vi "Rect Edit.vi"() -> ()   [LabVIEW 2013]
uses:
  Global Variables.vi
panel:
  in  "Index":i32=8
  in  "Direction":u16(ring) items=["Forward", "Backward"]
  in  "Enabled":bool=TRUE
  in  "Voltage Schedule":u16(ring) items=["Constant", "Ramp", "Fn. Generator", "Formula"]
  in  "Apply to All":bool
  in  "Fill Orientation":u16(ring) items=["Horizontal", "Vertical"]
  in  "Speed Schedule":u16(ring) items=["Constant", "Ramp", "Fn. Generator", "Formula"]
  in  "Speed (µm/s)":dbl=8.0
  in  "Voltage (V)":dbl=8.0
  in  "Speed Settings":bool
  in  "Voltage Settings":bool
  in  "Fill Spacing":dbl=0.1
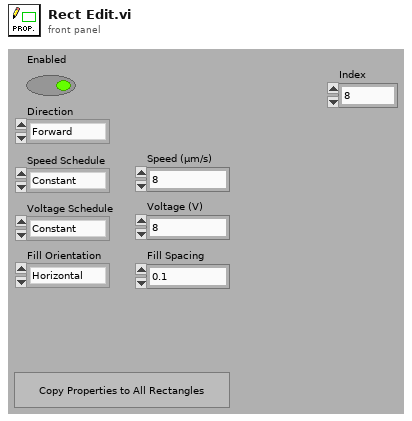
[diagram p1: front panel]
types:
  T1 = enum32{"invalid app kind", "Development System", "Run Time System", "Student Edition", "Embedded LabVIEW", "Evaluation", "Custom"}
  T2 = enum32{"Invalid", "Standard", "Closed", "Hidden", "Minimized", "Maximized"}
  T3 = cluster{"Enabled":bool, "Direction":u16, "Fill Orientation":u16, "Fill Spacing":dbl, "Speed (µm/s)":cluster{"Schedule":u16, "Value":dbl, "Start Value":dbl, "End Value":dbl, "Min Value":dbl, "Max Value":dbl, "Duty Cycle (%)":dbl, "Signal Type":u16, "Cycle Number":dbl, "Phase (degrees)":dbl}, "Voltage (V)":cluster{"Schedule":u16, "Value":dbl, "Start Value":dbl, "End Value":dbl, "Min Value":dbl, "Max Value":dbl, "Duty Cycle (%)":dbl, "Signal Type":u16, "Cycle Number":dbl, "Phase (degrees)":dbl}}[]
  T4 = cluster{"Enabled":bool, "Direction":u16, "Fill Orientation":u16, "Fill Spacing":dbl, "Speed (µm/s)":cluster{"Schedule":u16, "Value":dbl, "Start Value":dbl, "End Value":dbl, "Min Value":dbl, "Max Value":dbl, "Duty Cycle (%)":dbl, "Signal Type":u16, "Cycle Number":dbl, "Phase (degrees)":dbl}, "Voltage (V)":cluster{"Schedule":u16, "Value":dbl, "Start Value":dbl, "End Value":dbl, "Min Value":dbl, "Max Value":dbl, "Duty Cycle (%)":dbl, "Signal Type":u16, "Cycle Number":dbl, "Phase (degrees)":dbl}}
  T5 = cluster{"Schedule":u16, "Value":dbl, "Start Value":dbl, "End Value":dbl, "Min Value":dbl, "Max Value":dbl, "Duty Cycle (%)":dbl, "Signal Type":u16, "Cycle Number":dbl, "Phase (degrees)":dbl}
  T6 = cluster{"Schedule":u16, "Value":dbl, "Start Value":dbl, "End Value":dbl, "Min Value":dbl, "Max Value":dbl, "Duty Cycle (%)":dbl, "Speed Signal Type":u16, "Cycle Number":dbl, "Phase (degrees)":dbl}
  T7 = cluster{"Core":cluster{"Current VI Reference":refnum<vi>, "Close Panel on Exit?":bool}}
  T8 = cluster{"Current VI Reference":refnum<vi>, "Close Panel on Exit?":bool}
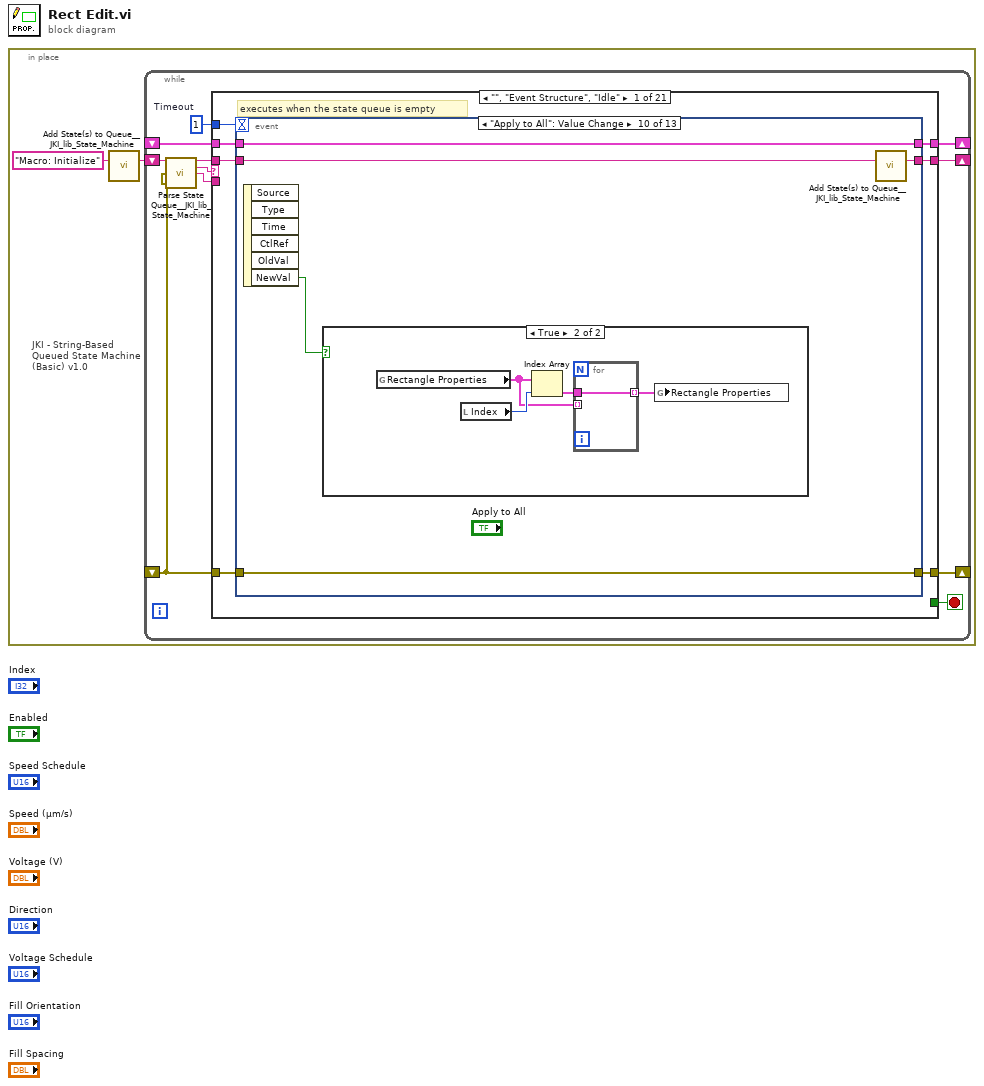
[diagram p0: block diagram]
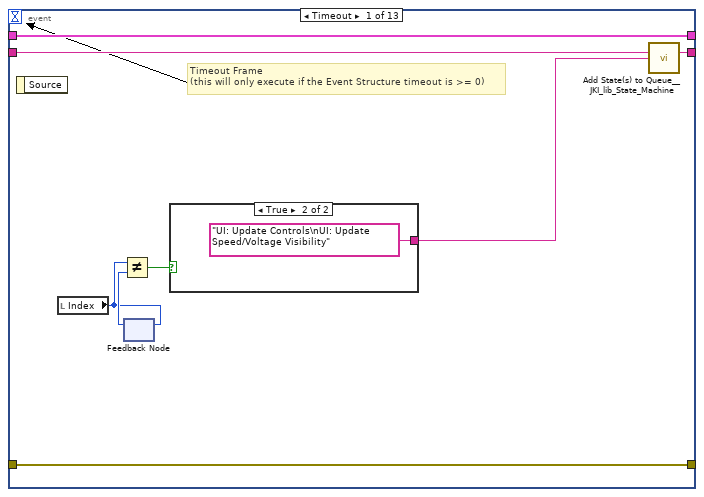
[diagram p2: hidden frame]
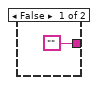
[diagram p3: hidden frame]
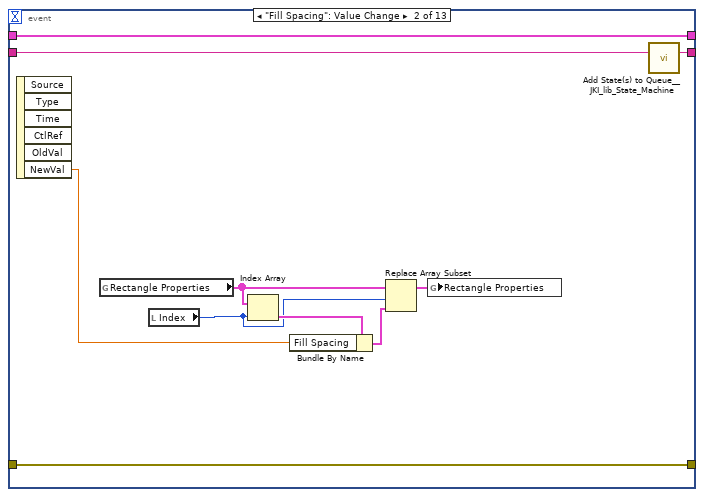
[diagram p4: hidden frame]
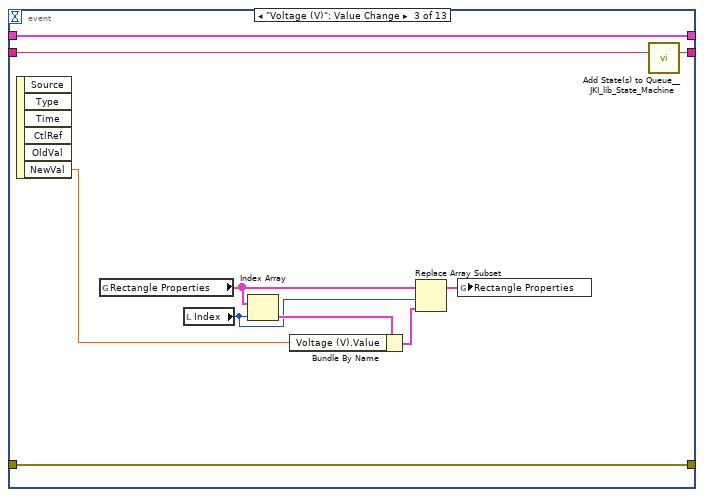
[diagram p5: hidden frame]
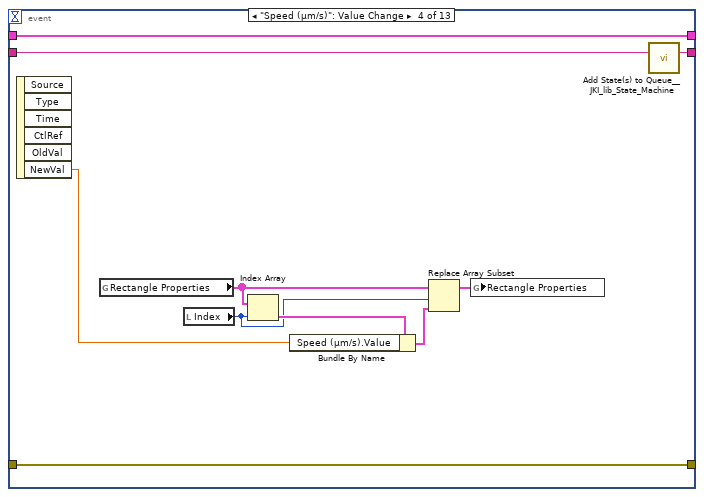
[diagram p6: hidden frame]
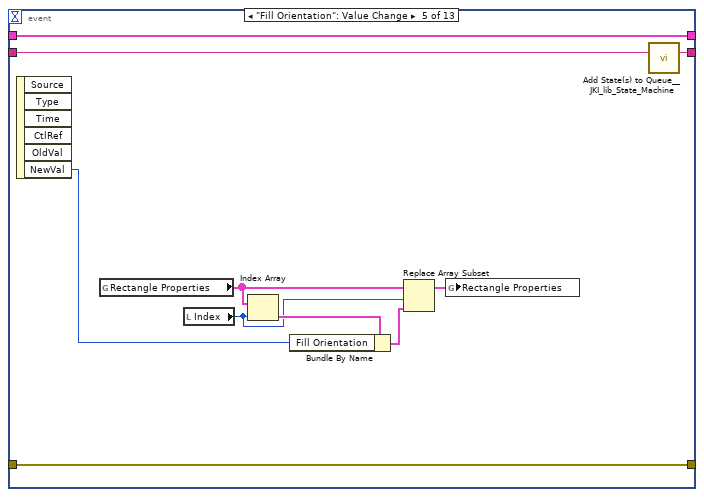
[diagram p7: hidden frame]
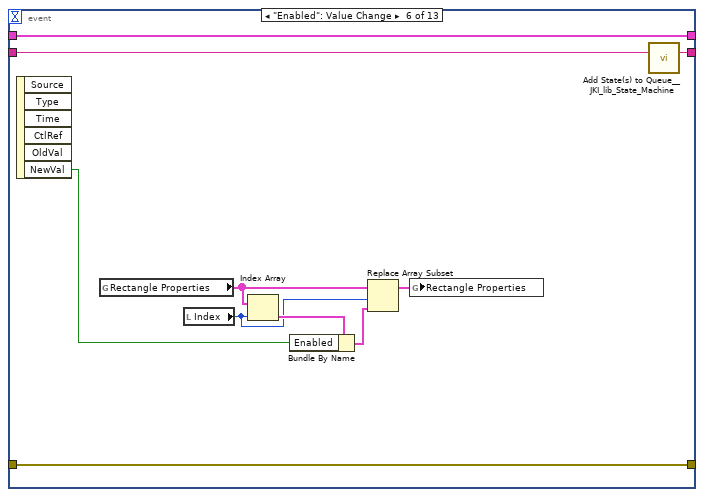
[diagram p8: hidden frame]
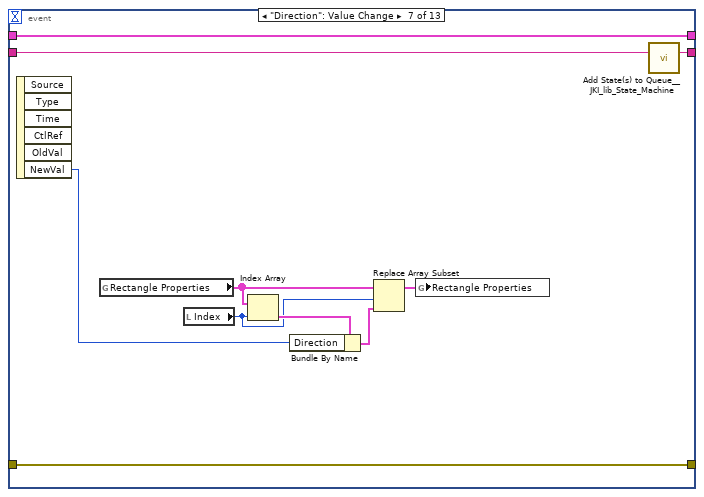
[diagram p9: hidden frame]
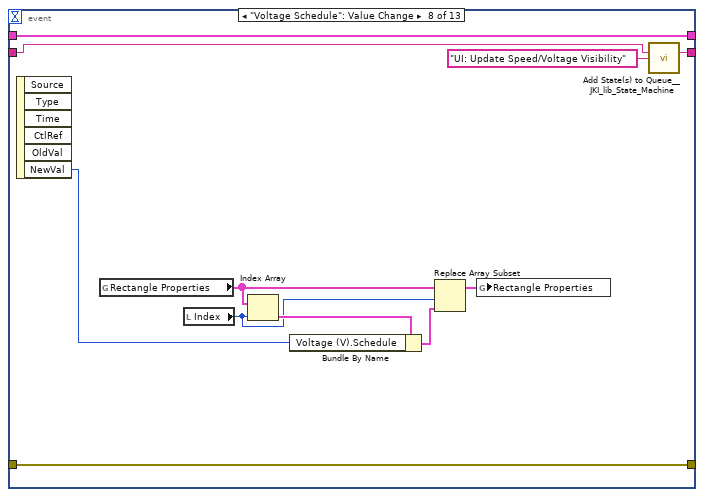
[diagram p10: hidden frame]
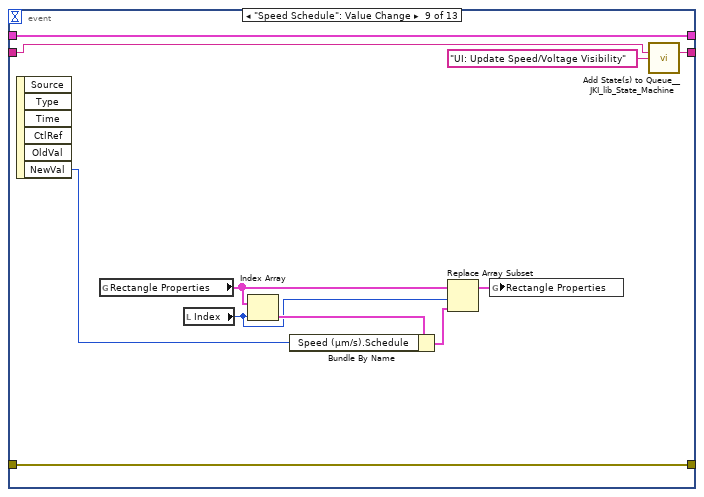
[diagram p11: hidden frame]
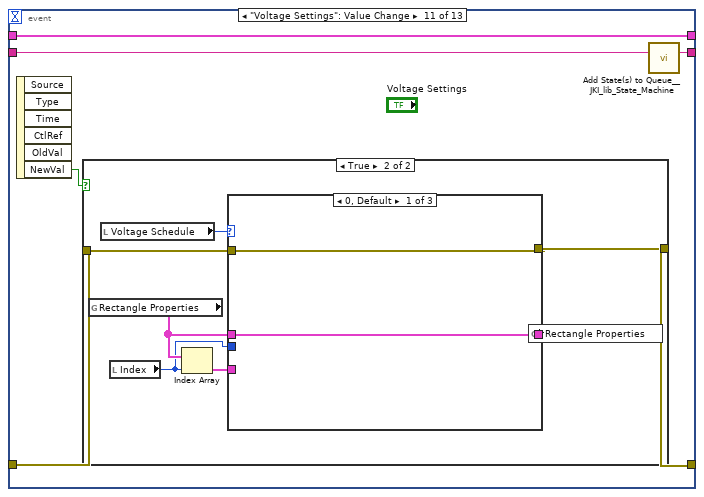
[diagram p13: hidden frame]
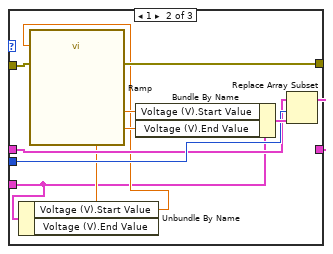
[diagram p15: hidden frame]
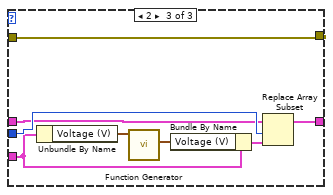
[diagram p16: hidden frame]
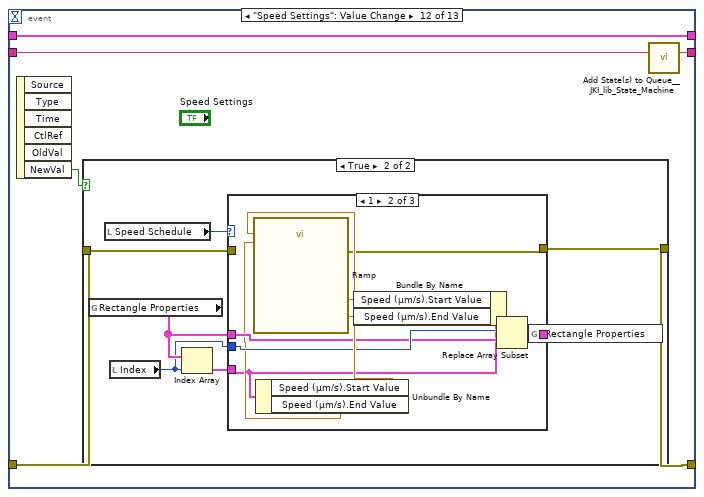
[diagram p17: hidden frame]
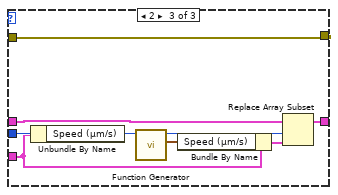
[diagram p20: hidden frame]
diagram:
  n1 = in-place {
    n2 = call <vilib>:"Add State(s) to Queue__JKI_lib_State_Machine.vi"("State(s) in (\"\")"="Macro: Initialize") -> ("States Out"=w2:string)  [unwired: 14 in]
    n3 = while "JKI - String-Based Queued State Machine (Basic) v1.0" {
      shift-right: [w6] -> _
      shift-left: _ -> [w5]
      shift-right: [w9] -> _
      shift-left: _ -> [w3]
      shift-right: [w8] -> _
      shift-left: w2 -> [w10]
      stop <- w7 stop-if-true
      w4 = 1  # Timeout
      n4 = call <vilib>:"Parse State Queue__JKI_lib_State_Machine.vi"("State Queue"=w10, "Error In (no error)"=w3) -> ("Remaining States"=w12:string, "Current State"=w13:string, "Arguments"=w11:string)  [unwired: 11 in]
      n5 = case shown="\"\", \"Event Structure\", \"Idle\"" w13 {
        selector: w13 -> [_ _ w202 _ _ _ _ _ _ _ _ _ _ _ _ _ _ _ _ _ _]
        tunnel: w12 -> [w20 w201 w206 w224 w230 w235 w239 w244 w250 w254 w258 w273 w279 w297 w308 w334 w339 w349 w353 w357 w361]
        tunnel: w11 -> [_ _ _ _ _ _ _ _ _ _ _ _ w274 _ w302 _ _ _ _ _ _]
        tunnel: w5 -> [w18 w198 w204 w220 w227 w233 w236 _ w248 w251 w256 w271 w277 w295 w304 w331 w336 w346 w350 w354 w358]
        tunnel: [w17 w199 w208 w221 errorcluster {"status"=FALSE, "code"=0, "source"=""} ("error out") w232 w237 w240 w246 w252 w255 w260 w275 w284 w305 w332 w337 w347 w351 w355 w359] -> w9
        tunnel: w3 -> [w16 w199 w207 w221 w226 w232 w237 w240 w245 w252 w255 w260 w276 w294 w306 w332 w337 w347 w351 w355 w359]
        tunnel: [w19 w200 w205 w223 w229 w234 w238 w243 w249 w253 w257 w272 w278 w296 w307 w333 w338 w348 w352 w356 w360] -> w8
        tunnel: [_ _ _ _ _ TRUE _ _ _ _ _ _ _ _ _ _ _ _ _ _ _] -> w7
        tunnel: [w15 w198 w204 w222 w227 w233 w236 w242 w248 w251 w256 w271 w277 w295 w304 w331 w336 w346 w350 w354 w358] -> w6
        tunnel: w4 -> [w14 _ _ _ _ _ _ _ _ _ _ _ _ _ _ _ _ _ _ _ _]
        frame "", "Event Structure", "Idle" {
          # "executes when the state queue is empty"
          n6 = event shown="[9] \"Apply to All\": Value Change" {
            selector: _ -> [_ _ _ _ _ _ _ _ _ _ _ _ _]
            dyn-events: _ -> [_ _ _ _ _ _ _ _ _ _ _ _ _]
            timeout: w14 -> [_ _ _ _ _ _ _ _ _ _ _ _ _]
            tunnel: w20 -> [w28 w40 w50 w60 w70 w80 w90 w101 w112 w117 w128 w163 w197]
            tunnel: [w27 w39 w49 w59 w69 w79 w89 w100 w111 w116 w127 w162 w196] -> w19
            tunnel: w18 -> [w25 w38 w48 w58 w68 w78 w88 w99 w110 w115 w126 w161 w194]
            tunnel: [w26 w32 w42 w52 w62 w72 w82 w93 w104 w114 w124 w159 w195] -> w17
            tunnel: w16 -> [w26 w32 w42 w52 w62 w72 w82 w93 w104 w114 w125 w160 w195]
            tunnel: [w25 w38 w48 w58 w68 w78 w88 w99 w110 w115 w126 w161 w194] -> w15
            event Timeout {
              # "Timeout Frame\n(this will only execute if the Event Structure timeout is >= 0)"
              n7 = event-data() -> ()  [unwired: 1 in, 1 out]
              n8 = local read "Index"() -> (w21:i32)
              n9 = feedback #1() -> (w24:i32)  [unwired: 1 in]
              n10 = Not Equal?(x=w21, y=w24) -> (x != y?=w23:bool)
              n11 = feedback-in #1(w21) -> ()
              n12 = case shown="True" w23 {
                tunnel: ["" "UI: Update Controls\nUI: Update Speed/Voltage Visibility"] -> w22
                frame False {
                }
                frame True {
                }
              }
              n13 = call <vilib>:"Add State(s) to Queue__JKI_lib_State_Machine.vi"("State(s) in (\"\")"=w28, "State(s) at Back (\"\")"=w22) -> ("States Out"=w27:string)  [unwired: 13 in]
            }
            event "Fill Spacing": Value Change {
              n14 = event-data() -> ("NewVal"=w36:dbl)  [unwired: 1 in, 5 out]
              n15 = global read "Global Variables.vi" "Rectangle Properties"() -> (w34:T3)
              n16 = local read "Index"() -> (w31:i32)
              n17 = Index Array(array=w34, index=w31) -> (element=w37:T4)
              n18 = Bundle By Name(cluster=w37, "Fill Spacing"=w36) -> (w35:T4)
              n19 = Replace Array Subset(array=w34, new element=w35, index=w31) -> (w33:T3)
              n20 = global write "Global Variables.vi" "Rectangle Properties"(w33) -> ()
              n21 = call <vilib>:"Add State(s) to Queue__JKI_lib_State_Machine.vi"("State(s) in (\"\")"=w40) -> ("States Out"=w39:string)  [unwired: 14 in]
            }
            event "Voltage (V)": Value Change {
              n22 = event-data() -> ("NewVal"=w46:dbl)  [unwired: 1 in, 5 out]
              n23 = global read "Global Variables.vi" "Rectangle Properties"() -> (w44:T3)
              n24 = local read "Index"() -> (w41:i32)
              n25 = Index Array(array=w44, index=w41) -> (element=w47:T4)
              n26 = Bundle By Name(cluster=w47, "Voltage (V).Value"=w46) -> (w45:T4)
              n27 = Replace Array Subset(array=w44, new element=w45, index=w41) -> (w43:T3)
              n28 = global write "Global Variables.vi" "Rectangle Properties"(w43) -> ()
              n29 = call <vilib>:"Add State(s) to Queue__JKI_lib_State_Machine.vi"("State(s) in (\"\")"=w50) -> ("States Out"=w49:string)  [unwired: 14 in]
            }
            event "Speed (µm/s)": Value Change {
              n30 = event-data() -> ("NewVal"=w56:dbl)  [unwired: 1 in, 5 out]
              n31 = global read "Global Variables.vi" "Rectangle Properties"() -> (w54:T3)
              n32 = local read "Index"() -> (w51:i32)
              n33 = Index Array(array=w54, index=w51) -> (element=w57:T4)
              n34 = Bundle By Name(cluster=w57, "Speed (µm/s).Value"=w56) -> (w55:T4)
              n35 = Replace Array Subset(array=w54, new element=w55, index=w51) -> (w53:T3)
              n36 = global write "Global Variables.vi" "Rectangle Properties"(w53) -> ()
              n37 = call <vilib>:"Add State(s) to Queue__JKI_lib_State_Machine.vi"("State(s) in (\"\")"=w60) -> ("States Out"=w59:string)  [unwired: 14 in]
            }
            event "Fill Orientation": Value Change {
              n38 = event-data() -> ("NewVal"=w66:u16)  [unwired: 1 in, 5 out]
              n39 = global read "Global Variables.vi" "Rectangle Properties"() -> (w64:T3)
              n40 = local read "Index"() -> (w61:i32)
              n41 = Index Array(array=w64, index=w61) -> (element=w67:T4)
              n42 = Bundle By Name(cluster=w67, "Fill Orientation"=w66) -> (w65:T4)
              n43 = Replace Array Subset(array=w64, new element=w65, index=w61) -> (w63:T3)
              n44 = global write "Global Variables.vi" "Rectangle Properties"(w63) -> ()
              n45 = call <vilib>:"Add State(s) to Queue__JKI_lib_State_Machine.vi"("State(s) in (\"\")"=w70) -> ("States Out"=w69:string)  [unwired: 14 in]
            }
            event "Enabled": Value Change {
              n46 = event-data() -> ("NewVal"=w76:bool)  [unwired: 1 in, 5 out]
              n47 = global read "Global Variables.vi" "Rectangle Properties"() -> (w74:T3)
              n48 = local read "Index"() -> (w71:i32)
              n49 = Index Array(array=w74, index=w71) -> (element=w77:T4)
              n50 = Bundle By Name(cluster=w77, "Enabled"=w76) -> (w75:T4)
              n51 = Replace Array Subset(array=w74, new element=w75, index=w71) -> (w73:T3)
              n52 = global write "Global Variables.vi" "Rectangle Properties"(w73) -> ()
              n53 = call <vilib>:"Add State(s) to Queue__JKI_lib_State_Machine.vi"("State(s) in (\"\")"=w80) -> ("States Out"=w79:string)  [unwired: 14 in]
            }
            event "Direction": Value Change {
              n54 = event-data() -> ("NewVal"=w86:u16)  [unwired: 1 in, 5 out]
              n55 = global read "Global Variables.vi" "Rectangle Properties"() -> (w84:T3)
              n56 = local read "Index"() -> (w81:i32)
              n57 = Index Array(array=w84, index=w81) -> (element=w87:T4)
              n58 = Bundle By Name(cluster=w87, "Direction"=w86) -> (w85:T4)
              n59 = Replace Array Subset(array=w84, new element=w85, index=w81) -> (w83:T3)
              n60 = global write "Global Variables.vi" "Rectangle Properties"(w83) -> ()
              n61 = call <vilib>:"Add State(s) to Queue__JKI_lib_State_Machine.vi"("State(s) in (\"\")"=w90) -> ("States Out"=w89:string)  [unwired: 14 in]
            }
            event "Voltage Schedule": Value Change {
              n62 = event-data() -> ("NewVal"=w97:u16)  [unwired: 1 in, 5 out]
              n63 = global read "Global Variables.vi" "Rectangle Properties"() -> (w95:T3)
              n64 = local read "Index"() -> (w91:i32)
              n65 = Index Array(array=w95, index=w91) -> (element=w98:T4)
              n66 = Bundle By Name(cluster=w98, "Voltage (V).Schedule"=w97) -> (w96:T4)
              n67 = Replace Array Subset(array=w95, new element=w96, index=w91) -> (w94:T3)
              n68 = global write "Global Variables.vi" "Rectangle Properties"(w94) -> ()
              n69 = call <vilib>:"Add State(s) to Queue__JKI_lib_State_Machine.vi"("State(s) in (\"\")"=w101, "State(s) at Back (\"\")"="UI: Update Speed/Voltage Visibility" ("State(s) at Back (\"\")")) -> ("States Out"=w100:string)  [unwired: 13 in]
            }
            event "Speed Schedule": Value Change {
              n70 = event-data() -> ("NewVal"=w108:u16)  [unwired: 1 in, 5 out]
              n71 = global read "Global Variables.vi" "Rectangle Properties"() -> (w106:T3)
              n72 = local read "Index"() -> (w102:i32)
              n73 = Index Array(array=w106, index=w102) -> (element=w109:T4)
              n74 = Bundle By Name(cluster=w109, "Speed (µm/s).Schedule"=w108) -> (w107:T4)
              n75 = Replace Array Subset(array=w106, new element=w107, index=w102) -> (w105:T3)
              n76 = global write "Global Variables.vi" "Rectangle Properties"(w105) -> ()
              n77 = call <vilib>:"Add State(s) to Queue__JKI_lib_State_Machine.vi"("State(s) in (\"\")"=w112, "State(s) at Back (\"\")"="UI: Update Speed/Voltage Visibility" ("State(s) at Back (\"\")")) -> ("States Out"=w111:string)  [unwired: 13 in]
            }
            event "Apply to All": Value Change {
              n78 = event-data() -> ("NewVal"=w113:bool)  [unwired: 1 in, 5 out]
              n79 = case shown="True" w113 {
                frame False {
                }
                frame True {
                  n80 = global read "Global Variables.vi" "Rectangle Properties"() -> (w118:T3)
                  n81 = local read "Index"() -> (w121:i32)
                  n82 = Index Array(array=w118, index=w121) -> (element=w120:T4)
                  n83 = for {
                    tunnel: w120 -> [w122]
                    tunnel: [w122] -> w119 mode=indexing
                    tunnel: w118 -> [_] mode=indexing
                  }
                  n84 = global write "Global Variables.vi" "Rectangle Properties"(w119) -> ()
                }
              }
              n85 = call <vilib>:"Add State(s) to Queue__JKI_lib_State_Machine.vi"("State(s) in (\"\")"=w117) -> ("States Out"=w116:string)  [unwired: 14 in]
            }
            event "Voltage Settings": Value Change {
              n86 = event-data() -> ("NewVal"=w123:bool)  [unwired: 1 in, 5 out]
              n87 = case shown="True" w123 {
                tunnel: w125 -> [w129 w135]
                tunnel: [w129 w134] -> w124
                frame False {
                }
                frame True {
                  n88 = global read "Global Variables.vi" "Rectangle Properties"() -> (w131:T3)
                  n89 = local read "Voltage Schedule"() -> (w136:u16)
                  n90 = local read "Index"() -> (w130:i32)
                  n91 = Index Array(array=w131, index=w130) -> (element=w132:T4)
                  n92 = case shown="0, Default" w136 {
                    tunnel: w135 -> [w138 w149 w153]
                    tunnel: [w138 w142 w153] -> w134
                    tunnel: [w137 w143 w154] -> w133
                    tunnel: w132 -> [_ w139 w152]
                    tunnel: w131 -> [w137 w144 w155]
                    tunnel: w130 -> [_ w145 w156]
                    frame 0, Default {
                    }
                    frame 1 {
                      n93 = Unbundle By Name(w139) -> ("Voltage (V).Start Value"=w141:dbl, "Voltage (V).End Value"=w140:dbl)
                      n94 = call "Ramp.vi"("Start Value"=w141, "End Value"=w140, "error in (no error)"=w149) -> ("End Value"=w147:dbl, "Start Value"=w148:dbl, "error out"=w142:errorcluster)  [unwired: 13 in, 1 out]
                      n95 = Bundle By Name(cluster=w139, "Voltage (V).Start Value"=w148, "Voltage (V).End Value"=w147) -> (w146:T4)
                      n96 = Replace Array Subset(array=w144, new element=w146, index=w145) -> (w143:T3)
                    }
                    frame 2 {
                      n97 = Unbundle By Name(w152) -> ("Voltage (V)"=w150:T5)
                      n98 = call "Function Generator.vi"("Properties in"=w150) -> ("Properties out"=w151:T6)  [unwired: 9 in, 1 out]
                      n99 = Bundle By Name(cluster=w152, "Voltage (V)"=w151) -> (w157:T4)
                      n100 = Replace Array Subset(array=w155, new element=w157, index=w156) -> (w154:T3)
                    }
                  }
                  n101 = global write "Global Variables.vi" "Rectangle Properties"(w133) -> ()
                }
              }
              n102 = call <vilib>:"Add State(s) to Queue__JKI_lib_State_Machine.vi"("State(s) in (\"\")"=w128) -> ("States Out"=w127:string)  [unwired: 14 in]
            }
            event "Speed Settings": Value Change {
              n103 = event-data() -> ("NewVal"=w158:bool)  [unwired: 1 in, 5 out]
              n104 = case shown="True" w158 {
                tunnel: w160 -> [w164 w170]
                tunnel: [w164 w169] -> w159
                frame False {
                }
                frame True {
                  n105 = global read "Global Variables.vi" "Rectangle Properties"() -> (w166:T3)
                  n106 = local read "Speed Schedule"() -> (w171:u16)
                  n107 = local read "Index"() -> (w165:i32)
                  n108 = Index Array(array=w166, index=w165) -> (element=w167:T4)
                  n109 = case shown="1" w171 {
                    tunnel: w170 -> [w173 _ w187]
                    tunnel: [w173 w179 w187] -> w169
                    tunnel: [w172 w178 w188] -> w168
                    tunnel: w167 -> [_ w174 w186]
                    tunnel: w166 -> [w172 w176 w189]
                    tunnel: w165 -> [_ w177 w190]
                    frame 0, Default {
                    }
                    frame 1 {
                      n110 = Unbundle By Name(w174) -> ("Speed (µm/s).Start Value"=w180:dbl, "Speed (µm/s).End Value"=w175:dbl)
                      n111 = call "Ramp.vi"("Start Value"=w180, "End Value"=w175) -> ("End Value"=w182:dbl, "Start Value"=w183:dbl, "error out"=w179:errorcluster)  [unwired: 14 in, 1 out]
                      n112 = Bundle By Name(cluster=w174, "Speed (µm/s).Start Value"=w183, "Speed (µm/s).End Value"=w182) -> (w181:T4)
                      n113 = Replace Array Subset(array=w176, new element=w181, index=w177) -> (w178:T3)
                    }
                    frame 2 {
                      n114 = Unbundle By Name(w186) -> ("Speed (µm/s)"=w184:T5)
                      n115 = call "Function Generator.vi"("Properties in"=w184) -> ("Properties out"=w185:T6)  [unwired: 9 in, 1 out]
                      n116 = Bundle By Name(cluster=w186, "Speed (µm/s)"=w185) -> (w191:T4)
                      n117 = Replace Array Subset(array=w189, new element=w191, index=w190) -> (w188:T3)
                    }
                  }
                  n118 = global write "Global Variables.vi" "Rectangle Properties"(w168) -> ()
                }
              }
              n119 = call <vilib>:"Add State(s) to Queue__JKI_lib_State_Machine.vi"("State(s) in (\"\")"=w163) -> ("States Out"=w162:string)  [unwired: 14 in]
            }
            event Panel Close? {
              # "Discard the event because we'll close the front panel ourselves in Macro: Exit"
              # "Close Panel button (pressed) Event\n(this executes Macro: Exit to terminate the VI)"
              n120 = event-data() -> ()  [unwired: 1 in, 1 out]
              n121 = event-data("Discard?"=TRUE) -> ()  [unwired: 1 in, 1 out]
              n122 = call <vilib>:"Add State(s) to Queue__JKI_lib_State_Machine.vi"("State(s) in Front (\"\")"="Macro: Exit", "State(s) in (\"\")"=w197) -> ("States Out"=w196:string)  [unwired: 13 in]
            }
          }
        }
        frame "---------- Core ----------" {
          # "Do not put any code in this frame.\n(it is a separator no-op)"
          n123 = call <vilib>:"Add State(s) to Queue__JKI_lib_State_Machine.vi"("State(s) in (\"\")"=w201) -> ("States Out"=w200:string)  [unwired: 14 in]
        }
        frame Default {
          w211 = 42 items=["No error", "Argument error", "Memory is full", "Out of zone", "End of file", "File already open", "Generic file I/O error", "File not found", "File permission error", "Disk is full", "Duplicate path", "Too many files open", "System feature not enabled", "Resource file not found", "Cannot add resource", "Resource not found", "Image not found", "Image memory error", "Pen does not exist", "Config type invalid", "Config token not found", "Config parse error", "Config memory error", "Bad external code format", "Bad external code offset", "External code not present", "Null window", "Destroy window error", "Null menu", "Print aborted", "Bad print record", "Print driver error", "Windows error during printing", "Memory error during printing", "Print dialog error", "Generic print error", "Invalid device refnum", "Device not found", "Device parameter error", "Device unit error", "Cannot open device", "Device call aborted", "Generic error", "Cancelled by user", "Object ID too low", "Object ID too high", "Object not in heap", "Unknown heap", "Unknown object (invalid DefProc)", "Unknown object (DefProc not in table)", "Message out of range", "Invalid (null) method", "Unknown message", "Manager call not supported", "Bad address", "Network operation in progress", "Network operation timed out", "Connection is busy", "Network attribute not supported", "Network error", "Address in use", "System out of memory", "Connection aborted", "Connection refused", "Not connected", "Already connected", "Connection closed", "Initialization error (interapplication manager)", "Bad occurrence", "Wait on unbound occurrence handler", "Occurrence queue overflow", "Datalog type conflict", "Unused", "Unrecognized type (interapplication manager)", "Memory corrupt", "Failed to make temporary DLL", "Old CIN version", "Drag socket not found", "Failed to load drop-object", "Failed to register OLE object", "Failed to release OLE object", "Format specifier type mismatch", "Unknown format specifier", "Too few format specifiers", "Too many format specifiers", "Scan failed", "Newer CIN version", "Error converting to variant", "Runtime menu error", "Password tampered", "Variant attribute not found", "Incompatible variant data type", "Event data is not available", "Event Store is not present", "Occurrence is not found", "Event Queue is not created", "Event info is not available", "Refnum passed is NULL", "Error retrieving Class GUID", "Error retrieving CoClass GUID", "Error retrieving TypeLib GUID.", "Bad built application magic bytes.", "Specific driver is different from the specific driver associated with the Logical Name.", "There is no session opened to the class driver.", "Max Error", "MAX - Error with config objects", "MAX - Error loading configuration", "MAX - Group not supported"]
          # "Current State"
          # "Do not delete, rename, or modify this frame.\n(this is used to capture unhandled states and typos)"
          # "Handle mistyped state name (developer tool)"
          n124 = Format Into String(format string="Software Exception: Unhandled State \"%s\"." ("message"), error in=w207, w202) -> (resulting string=w210:string, error out=w209:errorcluster)  [unwired: 1 in]
          n125 = call <vilib>:"Error Cluster From Error Code.vi"("show call chain? (False)"=TRUE, "error in (no error)"=w209, "error message (\"\")"=w210, "error code (0)"=w211) -> ("error out"=w208:errorcluster)  [unwired: 5 in]
          n126 = call <vilib>:"Add State(s) to Queue__JKI_lib_State_Machine.vi"("State(s) in (\"\")"=w206) -> ("States Out"=w205:string)  [unwired: 14 in]
        }
        frame "Initialize Core Data" {
          # "exe?"
          # "If panel starts closed or is an EXE, then close it when we exit"
          # "Do not delete, rename, or modify this frame.\n(this is used to determine panel behavior on exit)"
          n127 = property class="VI"() -> ("Front Panel.Open"=w218:bool)  [unwired: 2 in, 2 out]
          n128 = property class="App"() -> ("App.Kind"=w217:T1)  [unwired: 2 in, 2 out]
          n129 = control-ref of="Current VI Reference"() -> (w219:refnum<vi>)
          n130 = Not(x=w218) -> (.not. x?=w215:bool)
          n131 = Equal?(x=w217, y=T1."Run Time System" ("Application:Kind")) -> (x = y?=w214:bool)
          n132 = Or(x=w215, y=w214) -> (x .or. y?=w213:bool)
          n133 = Bundle By Name(cluster=w220, "Core.Current VI Reference"=w219, "Core.Close Panel on Exit?"=w213) -> (w222:T7)
          n134 = call <vilib>:"Add State(s) to Queue__JKI_lib_State_Machine.vi"("State(s) in (\"\")"=w224) -> ("States Out"=w223:string)  [unwired: 14 in]
        }
        frame "Error Handler" {
          # "Unhandled Error -- Display it"
          # "Handle any errors here.\nYou can also output any states to clean-up after errors occur"
          # "Clear error"
          n135 = call <vilib>:"General Error Handler.vi"("error in (no error)"=w226) -> ()  [unwired: 10 in, 5 out]
          n136 = call <vilib>:"Add State(s) to Queue__JKI_lib_State_Machine.vi"("State(s) in Front (\"\")"="/* Post Error States", "State(s) in (\"\")"=w230) -> ("States Out"=w229:string)  [unwired: 13 in]
        }
        frame "Exit" {
          # "Do not put any code in this frame.\n(No errors that occur here will be handled.)"
          n137 = call <vilib>:"Add State(s) to Queue__JKI_lib_State_Machine.vi"("State(s) in (\"\")"=w235) -> ("States Out"=w234:string)  [unwired: 14 in]
        }
        frame "---------- Data ----------" {
          # "Do not put any code in this frame.\n(It is a separator no-op. You can make a copy of this frame to create a new Data frame)"
          n138 = call <vilib>:"Add State(s) to Queue__JKI_lib_State_Machine.vi"("State(s) in (\"\")"=w239) -> ("States Out"=w238:string)  [unwired: 14 in]
        }
        frame "Data: Initialize" {
          w241 = T8 {"Current VI Reference"=refnum, "Close Panel on Exit?"=FALSE}  # Core
          # "Initialize the shift-register data, here.\n(data names are defined by what you wire into the bundle function)"
          n139 = Bundle("Core"=w241) -> (w242:T7)  [unwired: 1 in]
          n140 = call <vilib>:"Add State(s) to Queue__JKI_lib_State_Machine.vi"("State(s) in (\"\")"=w244) -> ("States Out"=w243:string)  [unwired: 14 in]
        }
        frame "Data: Cleanup" {
          # "Cleanup any data and references, here.\n(this is called automatically, by the Macro: Exit)"
          n141 = Unbundle By Name(w248) -> ("Core.Current VI Reference"=w247:refnum<vi>)
          n142 = Close Reference(reference=w247, error in (no error)=w245) -> (error out=w246:errorcluster)
          n143 = call <vilib>:"Add State(s) to Queue__JKI_lib_State_Machine.vi"("State(s) in (\"\")"=w250) -> ("States Out"=w249:string)  [unwired: 14 in]
        }
        frame "---------- UI ----------" {
          # "Do not put any code in this frame.\n(It is a separator no-op. You can make a copy of this frame to create a new UI frame)"
          n144 = call <vilib>:"Add State(s) to Queue__JKI_lib_State_Machine.vi"("State(s) in (\"\")"=w254) -> ("States Out"=w253:string)  [unwired: 14 in]
        }
        frame "UI: Initialize" {
          # "Initialize the User Interface, here.\n(this is called automatically, by the Macro: Init)"
          n145 = call <vilib>:"Add State(s) to Queue__JKI_lib_State_Machine.vi"("State(s) in (\"\")"=w258) -> ("States Out"=w257:string)  [unwired: 14 in]
        }
        frame "UI: Update Controls" {
          n146 = global read "Global Variables.vi" "Rectangle Properties"() -> (w259:T3)
          n147 = local read "Index"() -> (w264:i32)
          n148 = Index Array(array=w259, index=w264) -> (element=w263:T4)
          n149 = Unbundle By Name(w263) -> ("Enabled"=w265:bool, "Direction"=w266:u16, "Fill Orientation"=w267:u16, "Fill Spacing"=w268:dbl, "Speed (µm/s).Schedule"=w262:u16, "Speed (µm/s).Value"=w269:dbl, "Voltage (V).Schedule"=w261:u16, "Voltage (V).Value"=w270:dbl)
          n150 = local write "Enabled"(w265) -> ()
          n151 = local write "Direction"(w266) -> ()
          n152 = local write "Fill Orientation"(w267) -> ()
          n153 = local write "Fill Spacing"(w268) -> ()
          n154 = local write "Speed Schedule"(w262) -> ()
          n155 = local write "Speed (µm/s)"(w269) -> ()
          n156 = local write "Voltage Schedule"(w261) -> ()
          n157 = local write "Voltage (V)"(w270) -> ()
          n158 = call <vilib>:"Add State(s) to Queue__JKI_lib_State_Machine.vi"("State(s) in (\"\")"=w273) -> ("States Out"=w272:string)  [unwired: 14 in]
        }
        frame "UI: Cursor Set" {
          # "Argument"
          # "Set and Unset Cursor Busy.\n(Usage: \"UI: Cursor Set >> Busy|Idle\")"
          n159 = case shown="\"Idle\", Default" w274 {
            tunnel: w276 -> [w281 w283]
            tunnel: [w280 w282] -> w275
            frame "Idle", Default {
              n160 = call <vilib>:"Unset Busy.vi"("error in (no error)"=w281) -> ("error out"=w280:errorcluster)  [unwired: 10 in]
            }
            frame "Busy" {
              n161 = call <vilib>:"Set Busy.vi"("error in (no error)"=w283) -> ("error out"=w282:errorcluster)  [unwired: 9 in, 1 out]
            }
          }
          n162 = call <vilib>:"Add State(s) to Queue__JKI_lib_State_Machine.vi"("State(s) in (\"\")"=w279) -> ("States Out"=w278:string)  [unwired: 14 in]
        }
        frame "UI: Update Speed/Voltage Visibility" {
          n163 = local read "Voltage Schedule"() -> (w293:u16)
          n164 = case shown="0" w293 {
            tunnel: [TRUE FALSE] -> w289
            frame 0 {
            }
            frame 1, Default {
            }
          }
          n165 = local read "Speed Schedule"() -> (w292:u16)
          n166 = property on="Voltage (V)" class="DigNum (strict)"(error in=w294, "Visible"=w289) -> (error out=w290:errorcluster)  [unwired: 1 in, 1 out]
          n167 = case shown="0" w292 {
            tunnel: [TRUE FALSE] -> w285
            frame 0 {
            }
            frame 1, Default {
            }
          }
          n168 = Not(x=w289) -> (.not. x?=w288:bool)
          n169 = property on="Voltage Settings" class="Bool"(error in=w290, "Visible"=w288) -> (error out=w287:errorcluster)  [unwired: 1 in, 1 out]
          n170 = property on="Speed (µm/s)" class="DigNum (strict)"(error in=w287, "Visible"=w285) -> (error out=w286:errorcluster)  [unwired: 1 in, 1 out]
          n171 = Not(x=w285) -> (.not. x?=w291:bool)
          n172 = property on="Speed Settings" class="Bool"(error in=w286, "Visible"=w291) -> (error out=w284:errorcluster)  [unwired: 1 in, 1 out]
          n173 = call <vilib>:"Add State(s) to Queue__JKI_lib_State_Machine.vi"("State(s) in (\"\")"=w297) -> ("States Out"=w296:string)  [unwired: 14 in]
        }
        frame "UI: Front Panel State" {
          # "Argument"
          # "Set Front Panel Open or Closed\n(Usage: \"UI: Front Panel State >> Open|Close\")"
          n174 = Unbundle By Name(w304) -> ("Core.Current VI Reference"=w303:refnum<vi>)
          n175 = case shown="\"Open\", Default" w302 {
            tunnel: w306 -> [w312 w325]
            tunnel: [w314 w326] -> w305
            tunnel: w303 -> [w313 w323]
            frame "Open", Default {
              n176 = property class="VI"(reference=w313, error in=w312) -> (reference out=w310:refnum<vi>, error out=w311:errorcluster, "Front Panel.Open"=w309:bool)
              n177 = case shown="False" w309 {
                tunnel: [w317 w320] -> w314
                tunnel: w311 -> [w316 w320]
                tunnel: w310 -> [w315 _]
                frame False {
                  n178 = invoke class="VI" method="FP.Open"(reference=w315, error in=w316, "Activate"=TRUE, "State"=T2."Standard") -> (error out=w317:errorcluster)  [unwired: 1 in, 4 out]
                }
                frame True {
                }
              }
            }
            frame "Close" {
              n179 = property class="VI"(reference=w323, error in=w325) -> (reference out=w322:refnum<vi>, error out=w324:errorcluster, "Front Panel.Open"=w321:bool)
              n180 = case shown="True" w321 {
                tunnel: [w327 w330] -> w326
                tunnel: w324 -> [w327 w329]
                tunnel: w322 -> [_ w328]
                frame False {
                }
                frame True {
                  n181 = invoke class="VI" method="FP.Close"(reference=w328, error in=w329) -> (error out=w330:errorcluster)  [unwired: 1 in, 2 out]
                }
              }
            }
          }
          n182 = call <vilib>:"Add State(s) to Queue__JKI_lib_State_Machine.vi"("State(s) in (\"\")"=w308) -> ("States Out"=w307:string)  [unwired: 14 in]
        }
        frame "---------- Macro ----------" {
          # "Do not put any code in this frame.\n(It is a separator no-op. You can make a copy of this frame to create a new Macro frame)"
          n183 = call <vilib>:"Add State(s) to Queue__JKI_lib_State_Machine.vi"("State(s) in (\"\")"=w334) -> ("States Out"=w333:string)  [unwired: 14 in]
        }
        frame "Macro: Initialize" {
          w335 = "Data: Initialize\nInitialize Core Data\nUI: Initialize\nUI: Update Controls\nUI: Update Speed/Voltage Visibility\nUI: Front Panel State >> Close"  # Data: Initialize Initialize Core Data UI: Initialize UI: Update Controls UI: Update Speed/Voltage Visibility UI: Front Panel State >> Close
          # "Initialization Macro\n(This is called once, when the VI starts)"
          n184 = call <vilib>:"Add State(s) to Queue__JKI_lib_State_Machine.vi"("State(s) in Front (\"\")"=w335, "State(s) in (\"\")"=w339) -> ("States Out"=w338:string)  [unwired: 13 in]
        }
        frame "Macro: Exit" {
          # "Exit Macro\n(This is called once, when the VI exits)"
          n185 = Unbundle By Name(w346) -> ("Core.Close Panel on Exit?"=w345:bool)
          n186 = Select(t="UI: Front Panel State >> Close", s=w345, f="") -> (s? t:f=w342:string)
          n187 = call <vilib>:"Add State(s) to Queue__JKI_lib_State_Machine.vi"("State(s) in (\"\")"=w342, "State(s) at Back (\"\")"="Data: Cleanup\nExit") -> ("States Out"=w340:string)  [unwired: 13 in]
          n188 = call <vilib>:"Add State(s) to Queue__JKI_lib_State_Machine.vi"("State(s) in Front (\"\")"=w340, "State(s) in (\"\")"=w349) -> ("States Out"=w348:string)  [unwired: 13 in]
        }
        frame "---------- New Category ----------" {
          # "Template Separator\n(You can make a copy of, or modify, this frame)"
          n189 = call <vilib>:"Add State(s) to Queue__JKI_lib_State_Machine.vi"("State(s) in (\"\")"=w353) -> ("States Out"=w352:string)  [unwired: 14 in]
        }
        frame "New Category: 1" {
          # "Your code here.\n(You can make a copy of, or modify, this frame)"
          n190 = call <vilib>:"Add State(s) to Queue__JKI_lib_State_Machine.vi"("State(s) in (\"\")"=w357) -> ("States Out"=w356:string)  [unwired: 14 in]
        }
        frame "New Category: 2" {
          # "Your code here.\n(You can make a copy of, or modify, this frame)"
          n191 = call <vilib>:"Add State(s) to Queue__JKI_lib_State_Machine.vi"("State(s) in (\"\")"=w361) -> ("States Out"=w360:string)  [unwired: 14 in]
        }
      }
    }
  }
